vi "LaserCOM.vi"(3 "buffer à écrire":string="V?", 5 "Nom de ressource VISA":refnum<visa-resource-name>) -> (0 "sortie d'erreur":errorcluster, 1 "buffer lu":string, 2 "Nom de ressource VISA en sortie":refnum<visa-resource-name>)   [LabVIEW 2011]
panel:
  out "MachineState":string="MachineState"
  in  "stop":bool
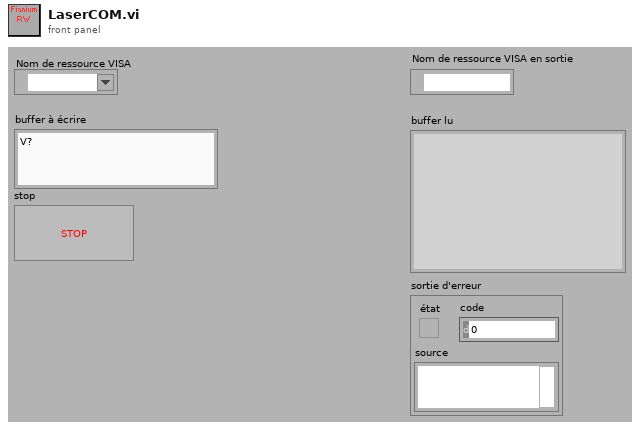
[diagram p1: front panel]
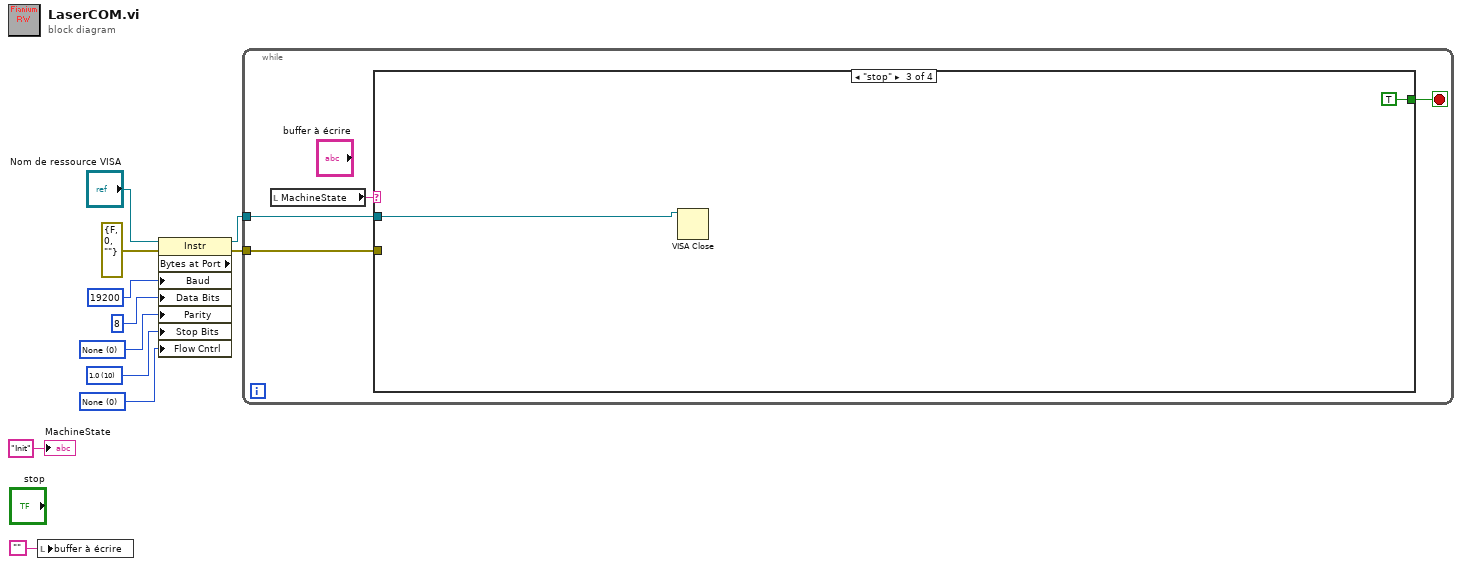
[diagram p0: block diagram]
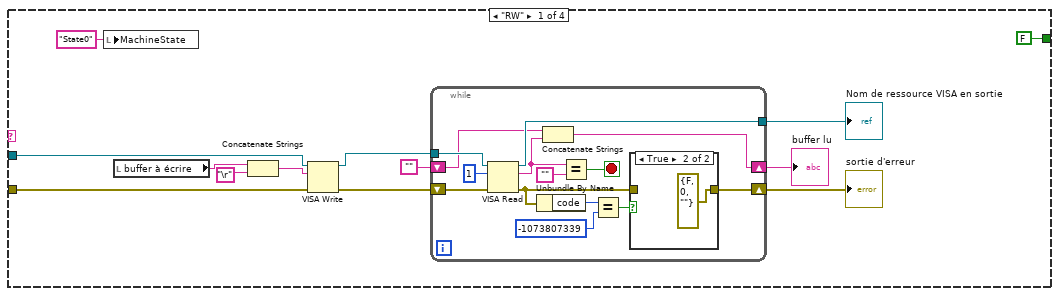
[diagram p2: hidden frame]
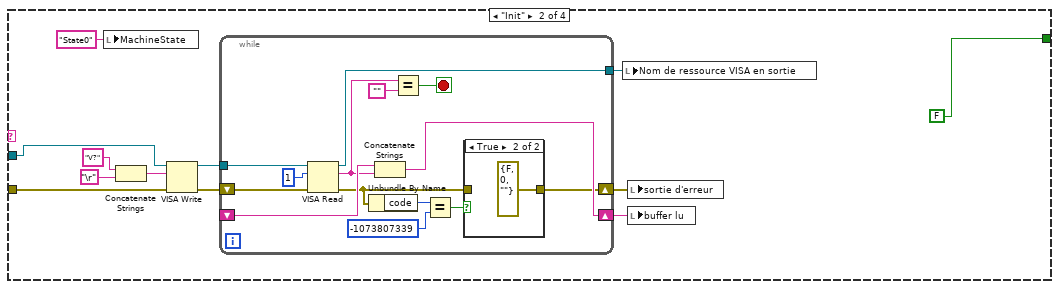
[diagram p4: hidden frame]
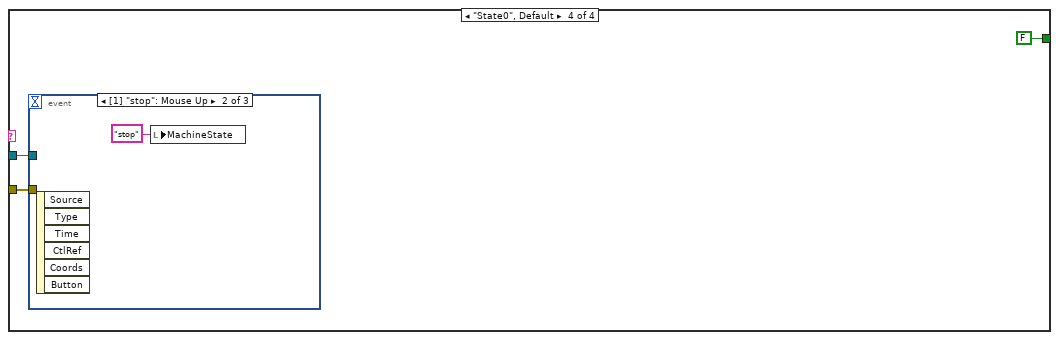
[diagram p6: hidden frame]
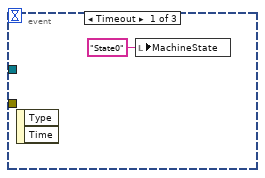
[diagram p7: hidden frame]
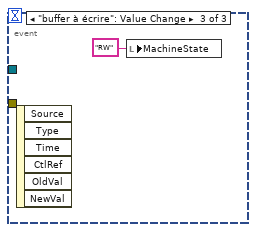
[diagram p8: hidden frame]
diagram:
  w7 = u16 0 items=["None", "XON/XOFF", "RTS/CTS", "XON/XOFF & RTS/CTS", "DTR/DSR", "XON/XOFF & DTR/DSR"] ("Serial Settings:Flow Control")
  w8 = u16 10 items=["1.0"=10, "1.5"=15, "2.0"=20] ("Serial Settings:Stop Bits")
  w9 = u16 0 items=["None", "Odd", "Even", "Mark", "Space"] ("Serial Settings:Parity")
  n1 = local write "buffer à écrire"("") -> ()
  n2 = property class="Instr" props=["Bytes at Port", "Baud", "Data Bits", "Parity", "Stop Bits", "Flow Cntrl"](reference="Nom de ressource VISA", error in=errorcluster {"status"=FALSE, "code"=0, "source"=""} ("entrée d'erreur (pas d'erreur)"), "Baud"=u32 19200 ("Serial Settings:Baud Rate"), "Data Bits"=u16 8 ("Serial Settings:Data Bits"), "Parity"=w9, "Stop Bits"=w8, "Flow Cntrl"=w7) -> (reference out=w4:refnum<visa-resource-name>, error out=w3:errorcluster)  [unwired: 1 out]
  n3 = while {
    tunnel: w4 -> [w15]
    tunnel: w3 -> [w14]
    stop <- w12 stop-if-true
    n4 = local read "MachineState"() -> (w13:string)
    n5 = case shown="\"stop\"" w13 {
      tunnel: w15 -> [w19 w55 w73 w77]
      tunnel: w14 -> [w18 w54 _ w76]
      tunnel: [FALSE FALSE TRUE FALSE] -> w12
      frame "RW" {
        n6 = local write "MachineState"("State0") -> ()
        n7 = local read "buffer à écrire"() -> (w21:string)
        n8 = Concatenate Strings(w21, "\r") -> (w20:string)
        n9 = VISA Write(VISA resource name=w19, write buffer=w20, error in (no error)=w18) -> (VISA resource name out=w26:refnum<visa-resource-name>, error out=w28:errorcluster)  [unwired: 1 out]
        n10 = while {
          tunnel: w26 -> [w42]
          tunnel: [w41] -> w24
          shift-right: [w35] -> w25
          shift-left: "" -> [w37]
          shift-right: [w29] -> w23
          shift-left: w28 -> [w34]
          stop <- w38 stop-if-true
          n11 = VISA Read(VISA resource name=w42, byte count=u32 1 ("nombre d'octets"), error in (no error)=w34) -> (VISA resource name out=w41:refnum<visa-resource-name>, read buffer=w36:string, error out=w30:errorcluster)  [unwired: 1 out]
          n12 = Unbundle By Name(w30) -> ("code"=w33:i32)
          n13 = Concatenate Strings(w37, w36) -> (w35:string)
          n14 = Equal?(x=w36, y="") -> (x = y?=w38:bool)
          n15 = Equal?(x=w33, y=-1073807339) -> (x = y?=w31:bool)
          n16 = case shown="True" w31 {
            tunnel: w30 -> [w43 _]
            tunnel: [w43 errorcluster {"status"=FALSE, "code"=0, "source"=""} ("entrée d'erreur (pas d'erreur)")] -> w29
            frame False {
            }
            frame True {
            }
          }
        }
        "buffer lu" <- w25
        "Nom de ressource VISA en sortie" <- w24
        "sortie d'erreur" <- w23
      }
      frame "Init" {
        n17 = local write "MachineState"("State0") -> ()
        n18 = Concatenate Strings("V?" ("chaîne"), "\r") -> (w47:string)
        n19 = VISA Write(VISA resource name=w55, write buffer=w47, error in (no error)=w54) -> (VISA resource name out=w50:refnum<visa-resource-name>, error out=w49:errorcluster)  [unwired: 1 out]
        n20 = while {
          tunnel: w50 -> [w57]
          tunnel: [w70] -> w53
          shift-right: [w64] -> w52
          shift-left: _ -> [w66]
          shift-right: [w58] -> w51
          shift-left: w49 -> [w63]
          stop <- w67 stop-if-true
          n21 = VISA Read(VISA resource name=w57, byte count=u32 1 ("nombre d'octets"), error in (no error)=w63) -> (VISA resource name out=w70:refnum<visa-resource-name>, read buffer=w65:string, error out=w59:errorcluster)  [unwired: 1 out]
          n22 = Unbundle By Name(w59) -> ("code"=w62:i32)
          n23 = Concatenate Strings(w66, w65) -> (w64:string)
          n24 = Equal?(x=w65, y="") -> (x = y?=w67:bool)
          n25 = Equal?(x=w62, y=-1073807339) -> (x = y?=w60:bool)
          n26 = case shown="True" w60 {
            tunnel: w59 -> [w71 _]
            tunnel: [w71 errorcluster {"status"=FALSE, "code"=0, "source"=""} ("entrée d'erreur (pas d'erreur)")] -> w58
            frame False {
            }
            frame True {
            }
          }
        }
        n27 = local write "Nom de ressource VISA en sortie"(w53) -> ()
        n28 = local write "sortie d'erreur"(w51) -> ()
        n29 = local write "buffer lu"(w52) -> ()
      }
      frame "stop" {
        n30 = VISA Close(VISA resource name=w73) -> ()  [unwired: 1 in, 1 out]
      }
      frame "State0", Default {
        n31 = event shown="[1] \"stop\": Mouse Up" {
          selector: _ -> [_ _ _]
          dyn-events: _ -> [_ _ _]
          timeout: _ -> [_ _ _]
          tunnel: w77 -> [_ _ _]
          tunnel: w76 -> [_ _ _]
          event Timeout {
            n32 = event-data() -> ()  [unwired: 3 out]
            n33 = local write "MachineState"("State0") -> ()
          }
          event "stop": Mouse Up {
            n34 = event-data() -> ()  [unwired: 7 out]
            n35 = local write "MachineState"("stop") -> ()
          }
          event "buffer à écrire": Value Change {
            n36 = event-data() -> ()  [unwired: 7 out]
            n37 = local write "MachineState"("RW") -> ()
          }
        }
      }
    }
  }
  "MachineState" <- "Init"
